vi "openDump.vi"(8 "error in":errorcluster, 11 "VISA resource name":refnum<visa-resource-name>="ASRL2::INSTR") -> (0 "error out":errorcluster, 3 "VISA resource out":refnum<visa-resource-name>="ASRL2::INSTR")   [LabVIEW 2010]
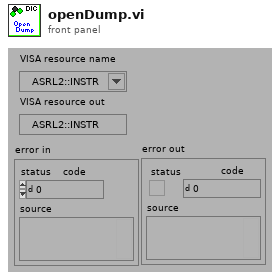
[diagram p1: front panel]
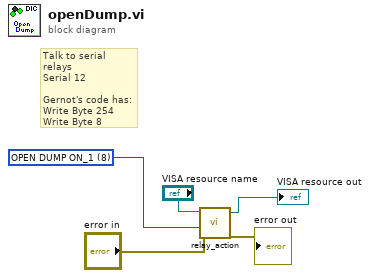
[diagram p0: block diagram]
diagram:
  w2 = u8 8 items=["OPEN DUMP ON_1"=8, "TurnON_PUMP"=9, "TurnON_3"=10, "TurnON_4"=11, "CLOSE DUMP OFF_1"=0, "TurnOFF_PUMP"=1, "TurnOFF_3"=2, "TurnOFF_4"=3, "OpenAll"=30, "CloseAllRelay"=29] ("Action")
  # "Talk to serial relays\nSerial 12\n\nGernot's code has: \nWrite Byte 254\nWrite Byte 8"
  n1 = call "relay_action.vi"("VISA resource in"="VISA resource name", "Action"=w2, "error in"="error in") -> ("VISA resource out"=→"VISA resource out":refnum<visa-resource-name>, "error out"=→"error out":errorcluster)  [unwired: 4 in]
